vi "QuitProcess.vi"(8 "error in":errorcluster caption="错误输入（无错误）", 10 "WDelay":u32=100, 11 "ComIn":refnum<visa-resource-name>) -> (0 "error out":errorcluster caption="错误输出", 1 "Times":u32, 3 "OK？":bool)   [LabVIEW 2013]
uses:
  <vilib>/Instr/_visa.llb/VISA Flush IO Buffer Mask.ctl
  <vilib>/Instr/_visa.llb/VISA Configure Serial Port (Instr).vi
panel:
  in  "Cycles":i32=5
  in  "Delay":u32=100
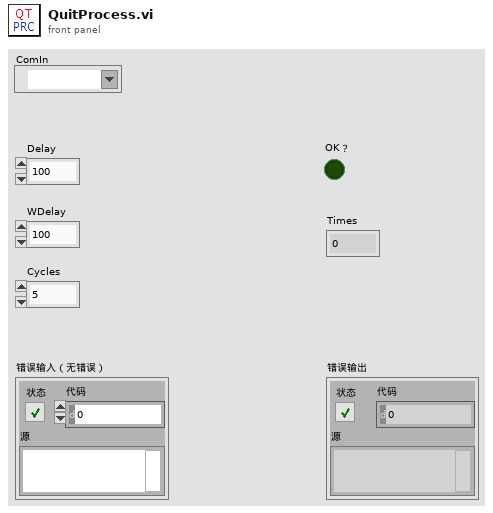
[diagram p1: front panel]
types:
  T1 = typedef "VISA Flush IO Buffer Mask.ctl" = u16
  T2 = cluster{"波特率":u32, "数据比特":u16, "奇偶":enum16{"None", "Odd", "Even", "Mark", "Space"}, "停止位":u16, "流控制":u16}
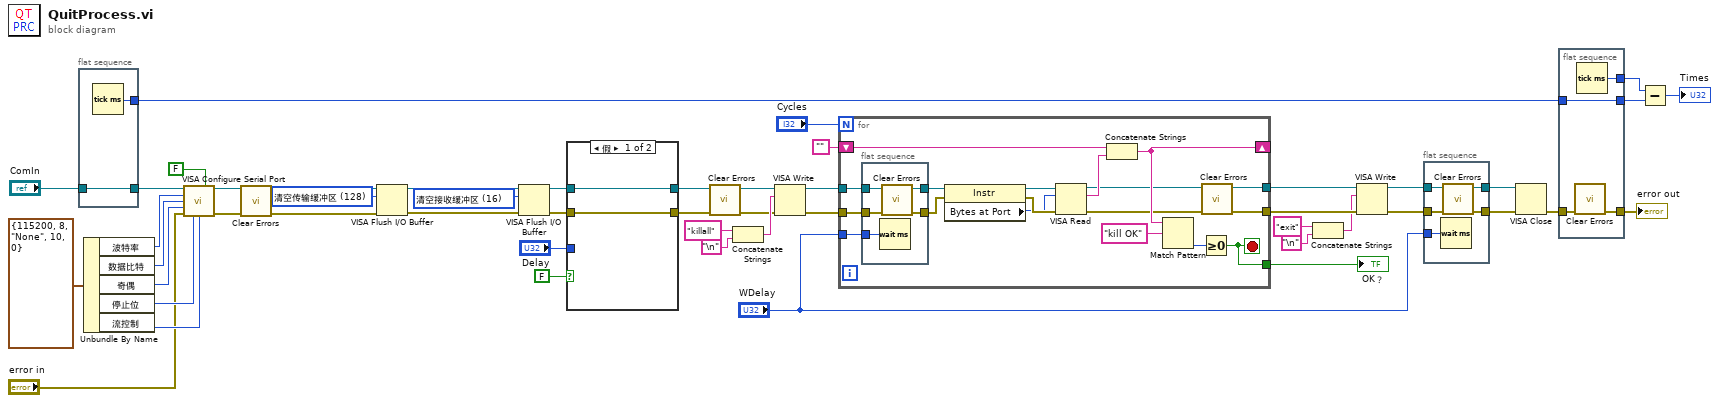
[diagram p0: block diagram]
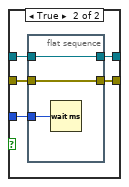
[diagram p2: hidden frame]
diagram:
  w36 = T1 16 items=["清空接收缓冲区"=16, "向设备写入传输缓冲区"=32, "清空接收缓冲区（无I/O）"=64, "清空传输缓冲区"=128] ("Mask")
  w39 = T1 128 items=["清空接收缓冲区"=16, "向设备写入传输缓冲区"=32, "清空接收缓冲区（无I/O）"=64, "清空传输缓冲区"=128] ("Mask")
  n1 = flat-sequence {
    tunnel: [w50] -> w10
    tunnel: "ComIn" -> [w50]
    tunnel: [w49] -> w5
    frame #0 {
      n2 = Tick Count (ms)() -> (millisecond timer value=w49:u32)
    }
  }
  n3 = Unbundle By Name(T2 {"波特率"=115200, "数据比特"=8, "奇偶"=enum."None", "停止位"=10, "流控制"=0} ("串口设置")) -> ("波特率"=w47:u32, "数据比特"=w46:u16, "奇偶"=w45:enum16{"None", "Odd", "Even", "Mark", "Space"}, "停止位"=w44:u16, "流控制"=w43:u16)
  n4 = call-poly "VISA Configure Serial Port"("VISA resource name"=w10, "Enable Termination\nChar (T)"=FALSE ("Enable Termination\nChar (T)"), "baud rate (9600)"=w47, "data bits (8)"=w46, "parity (0:none)"=w45, "error in (no error)"="error in", "stop bits (10: 1 bit)"=w44, "flow control (0:none)"=w43) -> ("VISA resource name out"=w41:refnum<visa-resource-name>, "error out"=w40:errorcluster)  [unwired: 6 in]
  n5 = call <vilib>:"Clear Errors.vi"("error in (no error)"=w40) -> ("error out"=w2:errorcluster)  [unwired: 6 in]
  n6 = VISA Flush I/O Buffer(VISA resource name=w41, mask (16)=w39, error in (no error)=w2) -> (VISA resource name out=w38:refnum<visa-resource-name>, error out=w37:errorcluster)
  n7 = VISA Flush I/O Buffer(VISA resource name=w38, mask (16)=w36, error in (no error)=w37) -> (VISA resource name out=w34:refnum<visa-resource-name>, error out=w32:errorcluster)
  n8 = case shown="假" FALSE {
    tunnel: [w52 w57] -> w35
    tunnel: w34 -> [w52 w56]
    tunnel: [w51 w55] -> w33
    tunnel: w32 -> [w51 w54]
    tunnel: "Delay" -> [_ w53]
    frame False {
    }
    frame True {
      n9 = flat-sequence {
        tunnel: [w60] -> w57
        tunnel: w56 -> [w60]
        tunnel: [w59] -> w55
        tunnel: w54 -> [w59]
        tunnel: w53 -> [w58]
        frame #0 {
          n10 = Wait (ms)(milliseconds to wait=w58) -> ()  [unwired: 1 out]
        }
      }
    }
  }
  n11 = call <vilib>:"Clear Errors.vi"("error in (no error)"=w33) -> ("error out"=w1:errorcluster)  [unwired: 6 in]
  n12 = Concatenate Strings("killall" ("写入缓冲区"), "\n") -> (w27:string)
  n13 = VISA Write(VISA resource name=w35, write buffer=w27, error in (no error)=w1) -> (VISA resource name out=w26:refnum<visa-resource-name>, error out=w25:errorcluster)  [unwired: 1 out]
  n14 = for {
    N: "Cycles" -> [_]
    tunnel: w26 -> [w77]
    tunnel: w25 -> [w76]
    shift-right: [w67] -> _
    shift-left: "" -> [w69]
    tunnel: "WDelay" -> [w73]
    tunnel: [w64] -> w17
    tunnel: [w63] -> w22
    tunnel: [w61] -> w21
    stop <- w64 stop-if-true
    n15 = flat-sequence {
      tunnel: w77 -> [w81]
      tunnel: [w81] -> w75
      tunnel: w76 -> [w80]
      tunnel: [w78] -> w74
      tunnel: w73 -> [w79]
      frame #0 {
        n16 = Wait (ms)(milliseconds to wait=w79) -> ()  [unwired: 1 out]
        n17 = call <vilib>:"Clear Errors.vi"("error in (no error)"=w80) -> ("error out"=w78:errorcluster)  [unwired: 6 in]
      }
    }
    n18 = property class="Instr"(reference=w75, error in=w74) -> (reference out=w70:refnum<visa-resource-name>, error out=w72:errorcluster, "Bytes at Port"=w71:u32)
    n19 = VISA Read(VISA resource name=w70, byte count=w71, error in (no error)=w72) -> (VISA resource name out=w63:refnum<visa-resource-name>, read buffer=w68:string, error out=w62:errorcluster)  [unwired: 1 out]
    n20 = Concatenate Strings(w69, w68) -> (w67:string)
    n21 = Match Pattern(string=w67, regular expression="kill OK" ("正则表达式")) -> (offset past match=w65:i32)  [unwired: 1 in, 3 out]
    n22 = Greater Or Equal To 0?(x=w65) -> (x >= 0?=w64:bool)
    n23 = call <vilib>:"Clear Errors.vi"("error in (no error)"=w62) -> ("error out"=w61:errorcluster)  [unwired: 6 in]
  }
  "OK？" <- w17
  n24 = Concatenate Strings("exit" ("写入缓冲区"), "\n") -> (w18:string)
  n25 = VISA Write(VISA resource name=w22, write buffer=w18, error in (no error)=w21) -> (VISA resource name out=w15:refnum<visa-resource-name>, error out=w14:errorcluster)  [unwired: 1 out]
  n26 = flat-sequence {
    tunnel: w15 -> [w85]
    tunnel: [w85] -> w11
    tunnel: w14 -> [w84]
    tunnel: [w82] -> w12
    tunnel: "WDelay" -> [w83]
    frame #0 {
      n27 = Wait (ms)(milliseconds to wait=w83) -> ()  [unwired: 1 out]
      n28 = call <vilib>:"Clear Errors.vi"("error in (no error)"=w84) -> ("error out"=w82:errorcluster)  [unwired: 6 in]
    }
  }
  n29 = VISA Close(VISA resource name=w11, error in (no error)=w12) -> (error out=w8:errorcluster)
  n30 = flat-sequence {
    tunnel: w8 -> [w89]
    tunnel: [w86] -> w7
    tunnel: [w88] -> w6
    tunnel: w5 -> [w87]
    tunnel: [w87] -> w4
    frame #0 {
      n31 = call <vilib>:"Clear Errors.vi"("error in (no error)"=w89) -> ("error out"=w86:errorcluster)  [unwired: 6 in]
      n32 = Tick Count (ms)() -> (millisecond timer value=w88:u32)
    }
  }
  n33 = Subtract(x=w6, y=w4) -> (x-y=→"Times":u32)
  "error out" <- w7
